vi "Keyence.Cmd.Connect.vi"(8 "error in (no error)":errorcluster, 9 "Timeout [ms] (1000)":i32=1000, 10 "IP":string) -> (0 "error out":errorcluster, 3 "connection ID out":refnum<k5>)   [LabVIEW 2016]
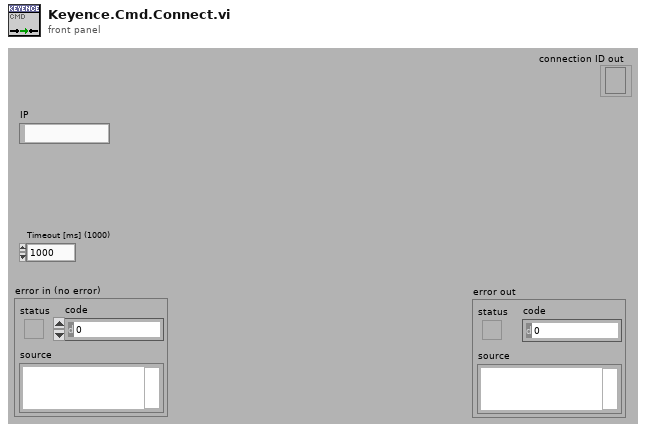
[diagram p1: front panel]
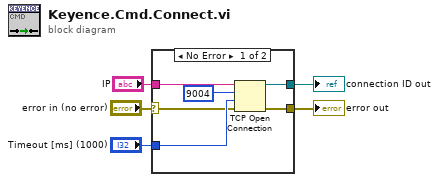
[diagram p0: block diagram]
diagram:
  n1 = case shown="No Error" "error in (no error)" {
    selector: "error in (no error)" -> [w10 w12]
    tunnel: "Timeout [ms] (1000)" -> [w11 _]
    tunnel: [w9 _] -> w3
    tunnel: [w8 w12] -> w2
    tunnel: "IP" -> [w6 _]
    frame No Error {
      n2 = TCP Open Connection(address=w6, remote port or service name=u16 9004 ("port"), timeout ms (60000)=w11, error in (no error)=w10) -> (connection ID=w9:refnum<k5>, error out=w8:errorcluster)  [unwired: 1 in]
    }
    frame Error {
    }
  }
  "error out" <- w2
  "connection ID out" <- w3
